vi "clone.vi"(0 "reference in":refnum<class "DQMHModuleNode.lvclass">, 5 "error in (no error)":errorcluster) -> (14 "reference out":refnum<class "DQMHModuleNode.lvclass">, 15 "clonedClassNode":refnum<class "AbstractNode.lvclass">, 19 "error out":errorcluster)   [LabVIEW 2016, in "DQMHModuleNode.lvclass"]
doc: "public Object clone()"
uses:
  <resource>/Framework/Providers/Open_GDS/UML/DQMHModuleNode_class/DQMHModuleNode.lvclass
  C:/Program Files (x86)/National Instruments/LabVIEW 2016/resource/Framework/Providers/Open_GDS/UML/AbstractNode_class/AbstractNode.lvclass
  <resource>/Framework/Providers/Open_GDS/UML/AbstractNode_class/AbstractNode.lvclass
  <resource>/Framework/Providers/Open_GDS/UML/MultiLineString_class/MultiLineString.lvclass
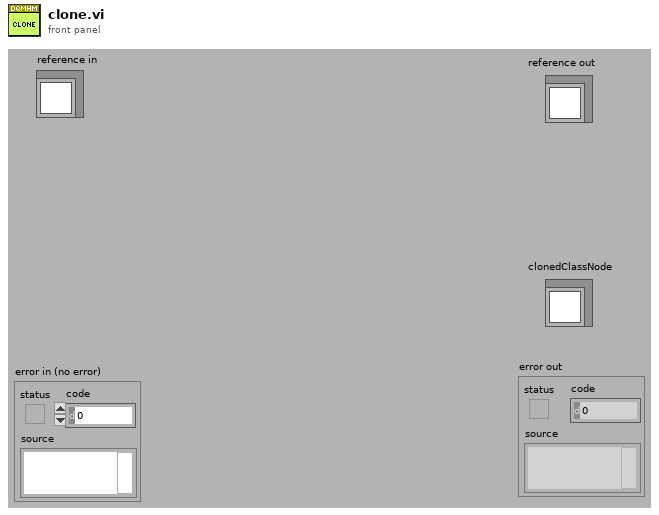
[diagram p1: front panel]
types:
  T1 = typedef "DQMHModuleNode.lvclass/ObjectAttributes.ctl" = cluster{"DescriptionHeight":dbl, "InternalDataHeight":dbl, "EventsHeight":dbl, "Name":refnum<class "MultiLineString.lvclass">, "Description":refnum<class "MultiLineString.lvclass">, "InternalData":refnum<class "MultiLineString.lvclass">, "Events":refnum<class "MultiLineString.lvclass">, "showDescription":bool, "showInternalData":bool, "showEvents":bool, "DEFAULT_ROUNDING":i32, "DEFAULT_WIDTH":i32, "DEFAULT_HEIGHT":i32, "ClassPath":path, "Template":string, "Icon":u8[][]}
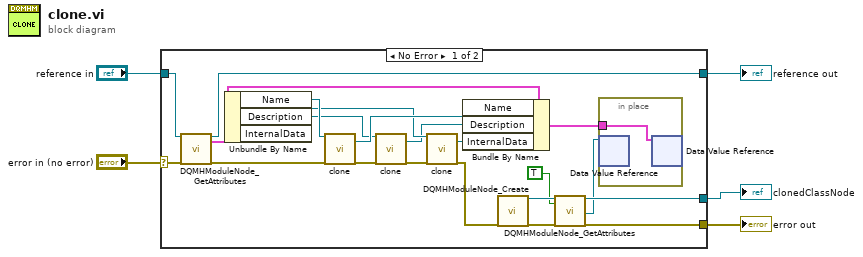
[diagram p0: block diagram]
diagram:
  n1 = case shown="No Error" "error in (no error)" {
    selector: "error in (no error)" -> [w25 w28]
    tunnel: "reference in" -> [w26 w29]
    tunnel: [w8 w28] -> w4
    tunnel: [w12 w29] -> w3
    tunnel: [w9 _] -> w1
    frame No Error {
      n2 = call <resource>:"DQMHModuleNode_GetAttributes.vi"("reference in"=w26, "error in (no error)"=w25) -> ("reference out"=w12:refnum<class "DQMHModuleNode.lvclass">, "Data"=w10:T1, "error out"=w16:errorcluster)  [unwired: 1 in, 14 out]
      n3 = Unbundle By Name(w10) -> ("Name"=w24:refnum<class "MultiLineString.lvclass">, "Description"=w20:refnum<class "MultiLineString.lvclass">, "InternalData"=w19:refnum<class "MultiLineString.lvclass">)
      n4 = call-dynamic "clone.vi"("reference"=w24, "error in (no error)"=w16) -> ("clonedMultiLineString"=w23:refnum<class "MultiLineString.lvclass">, "error out"=w22:errorcluster)  [unwired: 15 in, 1 out]
      n5 = call-dynamic "clone.vi"("reference"=w20, "error in (no error)"=w22) -> ("clonedMultiLineString"=w18:refnum<class "MultiLineString.lvclass">, "error out"=w21:errorcluster)  [unwired: 15 in, 1 out]
      n6 = call-dynamic "clone.vi"("reference"=w19, "error in (no error)"=w21) -> ("clonedMultiLineString"=w17:refnum<class "MultiLineString.lvclass">, "error out"=w13:errorcluster)  [unwired: 15 in, 1 out]
      n7 = Bundle By Name(cluster=w10, "Name"=w23, "Description"=w18, "InternalData"=w17) -> (w6:T1)
      n8 = call <resource>:"DQMHModuleNode_Create.vi"("error in (no error)"=w13) -> ("reference out"=w15:refnum<class "DQMHModuleNode.lvclass">, "error out"=w14:errorcluster)  [unwired: 17 in]
      n9 = call <resource>:"DQMHModuleNode_GetAttributes.vi"("reference in"=w15, "OnlyGetDvrReference(False)"=TRUE, "error in (no error)"=w14) -> ("reference out"=w9:refnum<class "DQMHModuleNode.lvclass">, "DataRef"=w7:refnum<data-value>, "error out"=w8:errorcluster)  [unwired: 13 in, 1 out]
      n10 = in-place {
        in-place-border: w6 -> [w27]
        n11 = in-place-dvr #1(w7) -> ()  [unwired: 2 out]
        n12 = in-place-dvr #1(w27) -> ()  [unwired: 2 out]
      }
    }
    frame Error {
    }
  }
  "reference out" <- w3
  "error out" <- w4
  "clonedClassNode" <- w1
